vi "Array of Single_ASCII String To Data.vi"(8 "error in (no error)":errorcluster, 9 "Default":cluster{"SGL Array":sgl[]}, 11 "Value":string) -> (0 "error out":errorcluster, 3 "Data":cluster{"SGL Array":sgl[]})   [LabVIEW 2020, in "Current Value Table(Rebuild).lvlib"]
doc: "This VI converts data stored on disk as an ascii string into the correct data type. This VI must perform the opposite operation to the DataToASCIIString function."
uses:
  Current Value Table(Rebuild).lvlib
  Errors/Generate Error.vi
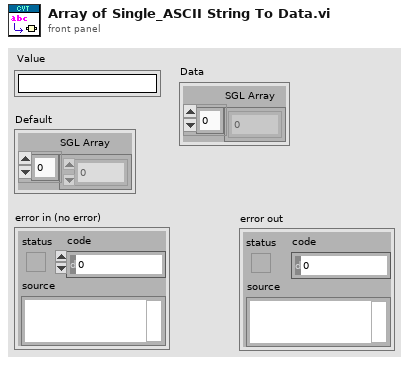
[diagram p1: front panel]
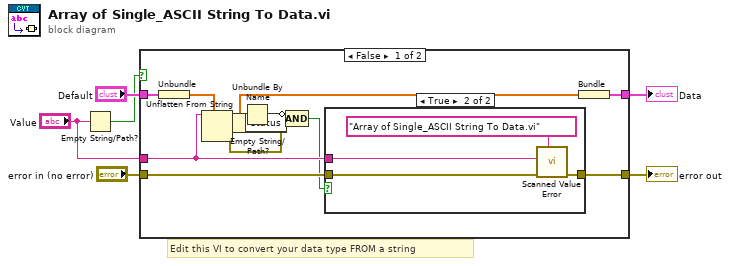
[diagram p0: block diagram]
diagram:
  # "Edit this VI to convert your data type FROM a string"
  n1 = Empty String/Path?(string/path="Value") -> (empty?=w3:bool)
  n2 = case shown="False" w3 {
    tunnel: "Default" -> [w16 w25]
    tunnel: "Value" -> [w12 _]
    tunnel: [w15 w25] -> w1
    tunnel: "error in (no error)" -> [w17 w24]
    tunnel: [w18 w24] -> w5
    frame False {
      n3 = Unbundle(w16) -> ("SGL Array"=w11:sgl[])
      n4 = Unflatten From String(type=w11, binary string=w12) -> (rest of the binary string=w10:string, value=w9:sgl[], error out=w13:errorcluster)  [unwired: 3 in]
      n5 = Unbundle By Name(w13) -> ("status"=w7:bool)
      n6 = Empty String/Path?(string/path=w10) -> (empty?=w14:bool)
      n7 = Compound Arithmetic op=AND(invert w14, w7) -> (w8:bool)
      n8 = case shown="True" w8 {
        tunnel: [w19 w23] -> w18
        tunnel: w17 -> [w19 w22]
        tunnel: w12 -> [_ w21]
        frame False {
        }
        frame True {
          n9 = call "Scanned Value Error.vi"("caller name"="Array of Single_ASCII String To Data.vi", "error in (no error)"=w22, "Value"=w21) -> ("error out"=w23:errorcluster)  [unwired: 8 in]
        }
      }
      n10 = Bundle("SGL Array"=w9) -> (w15:cluster{"SGL Array":sgl[]})  [unwired: 1 in]
    }
    frame True {
    }
  }
  "error out" <- w5
  "Data" <- w1
